vi "initialise_v2.vi"(0 "error in (no error)":errorcluster) -> (7 "error out":errorcluster, 8 "configuration":T1, 9 "network streaming queues":T2, 10 "FPGA VI Reference Out":refnum<k20>)   [LabVIEW 2010]
uses:
  network_streaming_queues_cluster.ctl
  scan_specification_cluster.ctl
  config_data_cluster.ctl
  <vilib>/userDefined/High Color/nirio_resource_hc.ctl
  <vilib>/rvi/interface/nirviOpenFPGA/nirviOpenFPGA.xnode
  FPGA Bitfiles/PCIe-7842R_main.lvbitx
  <vilib>/rvi/ClientSDK/nirviWhatTheDeviceIsDoing.ctl
  <vilib>/rvi/interface/nirviMethod/nirviMethod.xnode
  <vilib>/rvi/interface/nirviReadWriteControl/nirviReadWriteControl.xnode
  <vilib>/rvi/interface/common/niFpgaNodeNameForErrorReporting.ctl
  <vilib>/rvi/errors/niLvFpgaWhatHappensToTopLevelVI.ctl
  <vilib>/FPGAPlugInAG/PCIe-7842R/niLvFpga_Open_PCIe-7842R.vi
  <vilib>/rvi/interface/common/dynamic/niFpgaDynamicAddResources.vi
  <vilib>/Utility/error.llb/Error Cluster From Error Code.vi
  <vilib>/FPGAPlugInAG/Dynamic/niLvFpga_Reset_Dynamic.vi
  <vilib>/rvi/errors/niLvFpgaAdjustHostInterfaceError.vi
  NiFpgaLv.dll
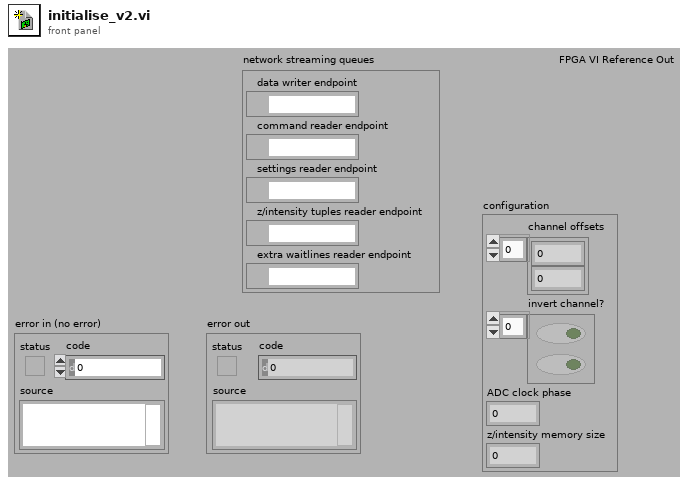
[diagram p1: front panel]
types:
  T1 = typedef "config_data_cluster.ctl" = cluster{"channel offsets":u32[], "invert channel?":bool[], "ADC clock phase":i32, "z/intensity memory size":i32}
  T2 = typedef "network_streaming_queues_cluster.ctl" = cluster{"data writer endpoint":refnum<k21>, "command reader endpoint":refnum<k21>, "settings reader endpoint":refnum<k21>, "z/intensity tuples reader endpoint":refnum<k21>, "extra waitlines reader endpoint":refnum<k21>}
  T3 = typedef "scan_specification_cluster.ctl" = cluster{"x amplitude":u16, "x resolution (pixels)":u16, "x offset fly-forward (iterations)":u16, "x offset fly-back (iterations)":u16, "y resolution (nr. of lines)":u16, "y step size":u16, "iterations per pixel":u16, "number of frames":i32, "y offset (pixels)":u16, "number of y-brake lines  (before y-fly-back)":u16, "number y-brake lines (after y-fly-back)":u16, "number of y-fly-back steps":u16, "lines per z step":u16, "number of z/intensity tuples":u16, "number of repetitions (volumes or planes)":i32, "z step size derived":u16, "choose the beginning of z scan":bool, "number of frames (settings)":i32, "FPGA trajectory?":bool, "Pockels cell voltage (bits)":i16, "Vy min(bits)":i16, "Vz min(bits)":i16}
  T4 = typedef "nirio_resource_hc.ctl" = tag
  T5 = typedef "niFpgaNodeNameForErrorReporting.ctl" = enum16{"Open FPGA VI Reference", "Read/Write Control", "Invoke Method: Abort", "Invoke Method: Acknowledge IRQ", "Invoke Method: Download", "Invoke Method: FIFO.Configure", "Invoke Method: FIFO.Read", "Invoke Method: FIFO.Start", "Invoke Method: FIFO.Stop", "Invoke Method: FIFO.Write", "Invoke Method: Reset", "Invoke Method: Run", "Invoke Method: Wait on IRQ", "Close FPGA VI Reference"}
  T6 = typedef "niLvFpgaWhatHappensToTopLevelVI.ctl" = enum16{"top level VI scripted behind XNode", "top level VI inlined behind XNode"}
  T7 = typedef "nirviWhatTheDeviceIsDoing.ctl" = enum32{"nothing", "something other than LabVIEW FPGA", "FPGA interface", "interactive", "emulation"}
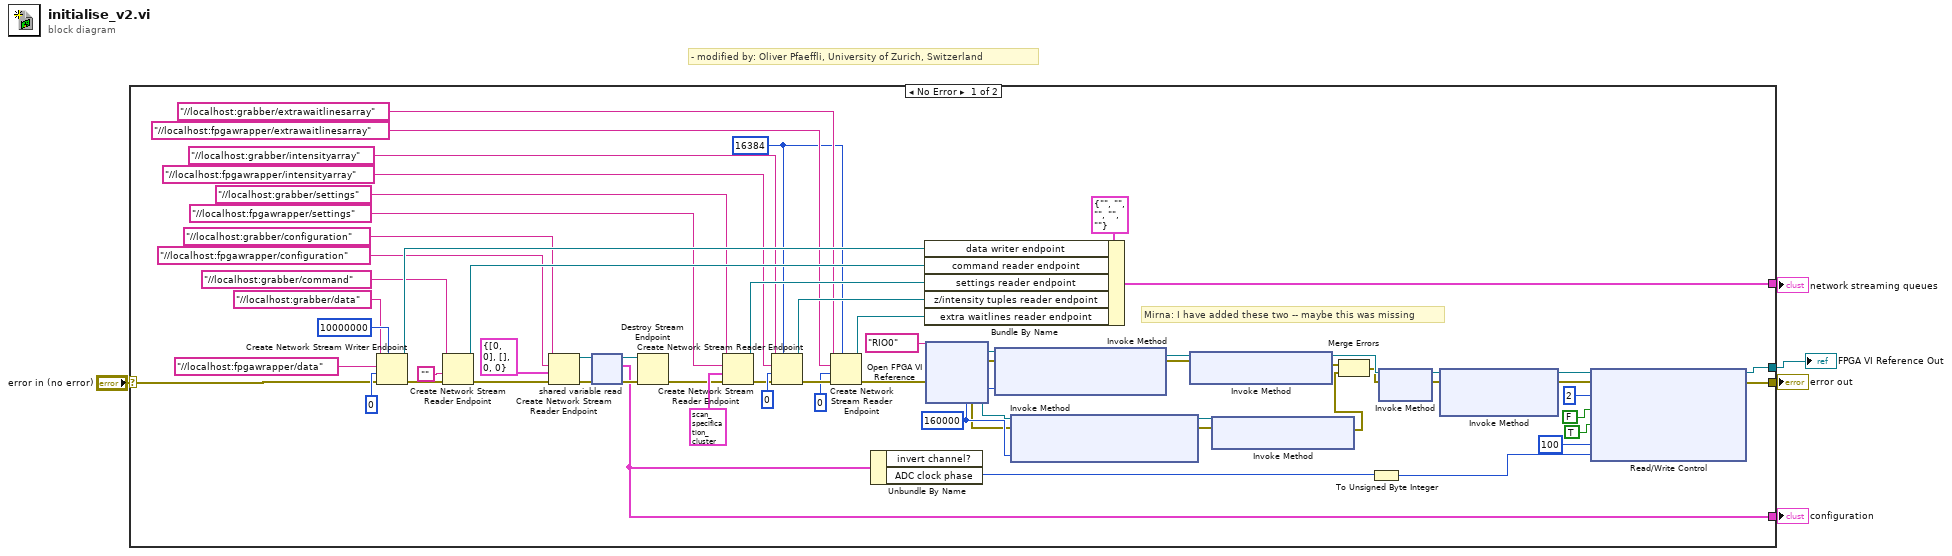
[diagram p0: block diagram]
diagram:
  # "- modified by: Oliver Pfaeffli, University of Zurich, Switzerland"
  n1 = case shown="No Error" "error in (no error)" {
    selector: "error in (no error)" -> [w40 w384]
    tunnel: [w39 w384] -> w4
    tunnel: [w60 _] -> w1
    tunnel: [w52 _] -> w3
    tunnel: [w38 _] -> w2
    frame No Error {
      w12 = u32 160000 ("Depth")
      w18 = 16384 ("reader buffer size")
      # "Mirna: I have added these two -- maybe this was missing"
      n2 = Create Network Stream Writer Endpoint(7:10000000 ("writer buffer size"), 8:w40, 9:u32 0, 10:"//localhost:fpgawrapper/data" ("reader url"), 11:"//localhost:grabber/data" ("writer name")) -> (0:w49:errorcluster, 3:w53:refnum<k21>)  [unwired: 1 in]
      n3 = Create Network Stream Reader Endpoint(8:w49, 9:"", 11:"//localhost:grabber/command" ("reader name")) -> (0:w25:errorcluster, 3:w48:refnum<k21>)  [unwired: 3 in]
      n4 = Create Network Stream Reader Endpoint(8:w25, 9:T1 {"channel offsets"=[0, 0], "invert channel?"=[], "ADC clock phase"=0, "z/intensity memory size"=0} ("configuration"), 10:"//localhost:fpgawrapper/configuration" ("writer name"), 11:"//localhost:grabber/configuration" ("reader name")) -> (0:w43:errorcluster, 3:w42:refnum<k21>)  [unwired: 2 in]
      n5 = shared-variable-read(w42, w43) -> (w41:refnum<k21>, w44:errorcluster, w38:T1)  [unwired: 1 in, 1 out]
      n6 = Destroy Stream Endpoint(8:w44, 11:w41) -> (0:w27:errorcluster)
      n7 = Create Network Stream Reader Endpoint(8:w27, 9:T3 {"x amplitude"=0, "x resolution (pixels)"=0, "x offset fly-forward (iterations)"=0, "x offset fly-back (iterations)"=0, "y resolution (nr. of lines)"=0, "y step size"=0, "iterations per pixel"=0, "number of frames"=0, "y offset (pixels)"=0, "number of y-brake lines  (before y-fly-back)"=0, "number y-brake lines (after y-fly-back)"=0, "number of y-fly-back steps"=0, "lines per z step"=0, "number of z/intensity tuples"=0, "number of repetitions (volumes or planes)"=0, "z step size derived"=0, "choose the beginning of z scan"=FALSE, "number of frames (settings)"=0, "FPGA trajectory?"=FALSE, "Pockels cell voltage (bits)"=0, "Vy min(bits)"=0, "Vz min(bits)"=0} ("scan specification"), 10:"//localhost:fpgawrapper/settings" ("writer name"), 11:"//localhost:grabber/settings" ("reader name")) -> (0:w26:errorcluster, 3:w32:refnum<k21>)  [unwired: 2 in]
      n8 = Create Network Stream Reader Endpoint(7:w18, 8:w26, 9:u32 0, 10:"//localhost:fpgawrapper/intensityarray" ("writer name"), 11:"//localhost:grabber/intensityarray" ("reader name")) -> (0:w24:errorcluster, 3:w28:refnum<k21>)  [unwired: 1 in]
      n9 = Create Network Stream Reader Endpoint(7:w18, 8:w24, 9:u32 0, 10:"//localhost:fpgawrapper/extrawaitlinesarray" ("writer name"), 11:"//localhost:grabber/extrawaitlinesarray" ("reader name")) -> (0:w23:errorcluster, 3:w19:refnum<k21>)  [unwired: 1 in]
      n10 = Unbundle By Name(w38) -> ("ADC clock phase"=w36:i32)  [unwired: 1 out]
      n11 = Bundle By Name(cluster=T2 {"data writer endpoint"="", "command reader endpoint"="", "settings reader endpoint"="", "z/intensity tuples reader endpoint"="", "extra waitlines reader endpoint"=""} ("network streaming queues"), "data writer endpoint"=w53, "command reader endpoint"=w48, "settings reader endpoint"=w32, "z/intensity tuples reader endpoint"=w28, "extra waitlines reader endpoint"=w19) -> (w52:T2)
      n12 = xnode "Open FPGA VI Reference"("error in"=w23, "resource name"=T4 "RIO0") -> ("FPGA VI Reference Out"=w11:refnum<k20>, "error out"=w10:errorcluster)
      n13 = xnode "Invoke Method"("FPGA VI Reference In"=w11, "error in"=w10, "Depth"=w12) -> ("FPGA VI Reference Out"=w16:refnum<k20>, "error out"=w15:errorcluster)
      n14 = xnode "Invoke Method"("FPGA VI Reference In"=w11, "error in"=w10, "Depth"=w12) -> ("FPGA VI Reference Out"=w9:refnum<k20>, "error out"=w8:errorcluster)
      n15 = xnode "Invoke Method"("FPGA VI Reference In"=w16, "error in"=w15) -> ("FPGA VI Reference Out"=w14:refnum<k20>, "error out"=w13:errorcluster)
      n16 = xnode "Invoke Method"("FPGA VI Reference In"=w9, "error in"=w8) -> ("error out"=w6:errorcluster)  [unwired: 1 out]
      n17 = Merge Errors(w13, w6) -> (w7:errorcluster)
      n18 = To Unsigned Byte Integer(number=w36) -> (unsigned 8bit integer=w17:u8)
      n19 = xnode "Invoke Method"("FPGA VI Reference In"=w14, "error in"=w7) -> ("FPGA VI Reference Out"=w64:refnum<k20>, "error out"=w63:errorcluster)
      n20 = xnode "Invoke Method"("FPGA VI Reference In"=w64, "error in"=w63) -> ("FPGA VI Reference Out"=w66:refnum<k20>, "error out"=w65:errorcluster)  [unwired: 1 out]
      n21 = xnode "Read/Write Control"("FPGA VI Reference In"=w66, "error in"=w65, "converter box version"=i16 2, "FIFO overflow"=FALSE, "enable fly-back reversion?"=TRUE, "sync minimum high"=i16 100, "ADC clock phase"=w17) -> ("FPGA VI Reference Out"=w60:refnum<k20>, "error out"=w39:errorcluster)
    }
    frame Error {
    }
  }
  "error out" <- w4
  "network streaming queues" <- w3
  "configuration" <- w2
  "FPGA VI Reference Out" <- w1
